vi "Write Pick and Place Type.vi"(8 "error in (no error)":errorcluster, 10 "Pick and Place Type":T1, 11 "Pick and Place in":refnum<class "Pick and Place.lvclass">) -> (0 "error out":errorcluster, 3 "Pick and Place out":refnum<class "Pick and Place.lvclass">)   [LabVIEW 2020, in "Pick and Place.lvclass"]
uses:
  Pick and Place.lvclass
  Pick and Place Type.ctl
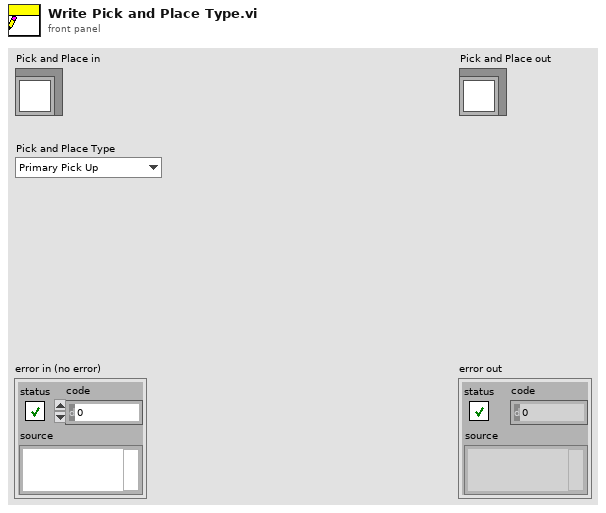
[diagram p1: front panel]
types:
  T1 = typedef "Pick and Place.lvclass/Pick and Place Type.ctl" = enum16{"Primary Pick Up", "Secondary Pick Up", "Put Down All", "Pick Up All", "Put Down Secondary"}
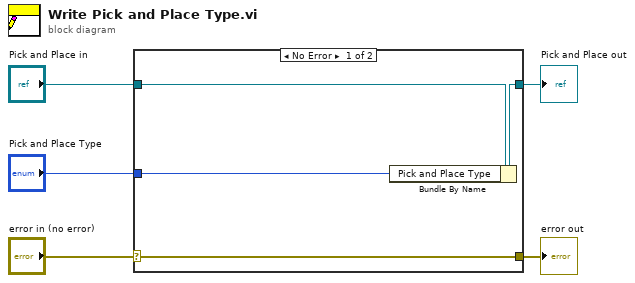
[diagram p0: block diagram]
diagram:
  n1 = case shown="No Error" "error in (no error)" {
    selector: "error in (no error)" -> [w9 w10]
    tunnel: [w9 w10] -> w4
    tunnel: [w7 w11] -> w2
    tunnel: "Pick and Place in" -> [w8 w11]
    tunnel: "Pick and Place Type" -> [w6 _]
    frame No Error {
      n2 = Bundle By Name(cluster=w8, "Pick and Place Type"=w6) -> (w7:refnum<class "Pick and Place.lvclass">)
    }
    frame Error {
    }
  }
  "error out" <- w4
  "Pick and Place out" <- w2
